vi "Inspect Tell Child.vi"(4 "Priority":bool, 6 "Reply":bool, 8 "Error in":errorcluster, 9 "Msg in":refnum<class "Msg.lvclass">, 10 "UID":string, 11 "Base Actor in":refnum<class "Base Actor.lvclass">) -> (0 "Error out":errorcluster, 1 "Msg out":refnum<class "Msg.lvclass">, 2 "Proceed":bool=TRUE, 3 "Base Actor out":refnum<class "Base Actor.lvclass">)   [LabVIEW 2020, in "jettl.lvlib" / "Base jettl Actor.lvlib" / "Base Actor.lvlib" / "Base Actor.lvclass"]
uses:
  Base Actor.lvclass
  Msg/Msg.lvclass
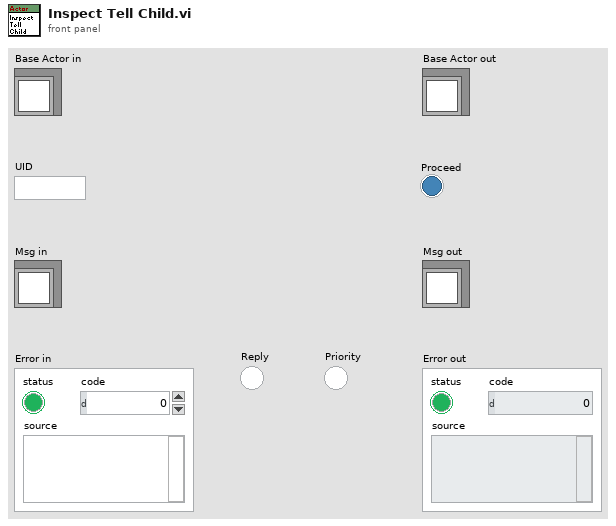
[diagram p1: front panel]
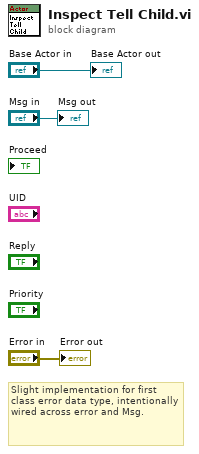
[diagram p0: block diagram]
diagram:
  # "Slight implementation for first class error data type, intentionally wired across error and Msg."
  "Base Actor out" <- "Base Actor in"
  "Error out" <- "Error in"
  "Msg out" <- "Msg in"
